vi "Change Screw Speed.vi"(8 "error in (no error)":errorcluster, 10 "Screw":u16(ring)=1 items=["0%"=1, "25%"=225, "50%"=450, "75%"=675, "100%"=900], 11 "Feeder Actor.lvlib:Screw.lvclass":refnum<class "Screw.lvclass">) -> (0 "error out":errorcluster, 3 "Actor out":refnum<class "Actor.lvclass">)   [LabVIEW 2018, in "Feeder Actor.lvlib" / "Screw.lvclass"]
uses:
  Screw.lvclass
  <vilib>/ActorFramework/Actor/Actor.lvclass
  C:/Program Files (x86)/National Instruments/LabVIEW 2018/vi.lib/ActorFramework/Actor/Actor.lvclass
  Screw.lvclass/Screw.ctl
  <vilib>/DAQmx/write.llb/DAQmx Write (Counter Frequency 1Chan 1Samp).vi
  <vilib>/DAQmx/miscellaneous.llb/DAQmx Fill In Error Info.vi
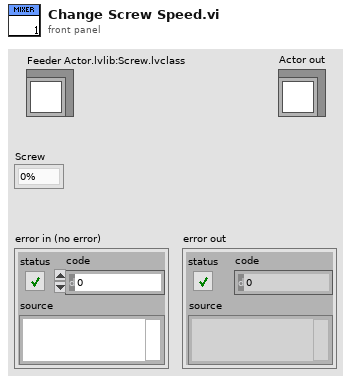
[diagram p1: front panel]
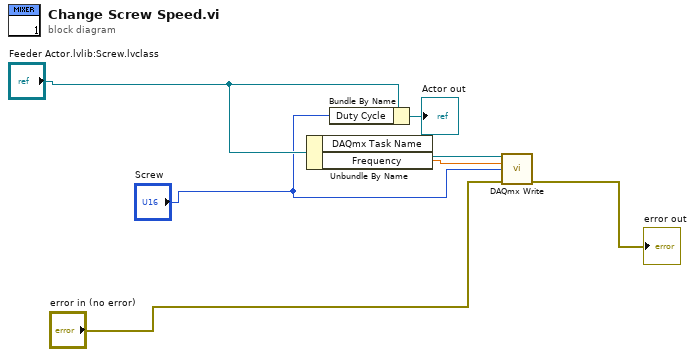
[diagram p0: block diagram]
diagram:
  n1 = Unbundle By Name("Feeder Actor.lvlib:Screw.lvclass") -> ("DAQmx Task Name"=w7:refnum<k21>, "Frequency"=w6:dbl)
  n2 = Bundle By Name(cluster="Feeder Actor.lvlib:Screw.lvclass", "Duty Cycle"="Screw") -> (→"Actor out":refnum<class "Screw.lvclass">)
  n3 = call-poly <vilib>:"DAQmx Write.vi"("task/channels in"=w7, "frequency"=w6, "duty cycle"="Screw", "error in"="error in (no error)") -> ("error out"=→"error out":errorcluster)  [unwired: 9 in, 2 out]
